vi "RunTest.vi"(8 "error in (no error)":errorcluster, 11 "TestCaseMock in":refnum<class "TestCaseMock.lvclass">) -> (0 "error out":errorcluster, 3 "TestCaseMock out":refnum<class "TestCaseMock.lvclass">)   [LabVIEW 2017, in "TestResultTest.lvlib" / "Support.lvlib" / "TestCaseMock.lvclass"]
doc: "Override to run the test and assert its state."
uses:
  TestCaseMock.lvclass
  Error/Error.lvlib
  a4c9ca4c-822c-43fa-bc73-5b07c458682f.vi
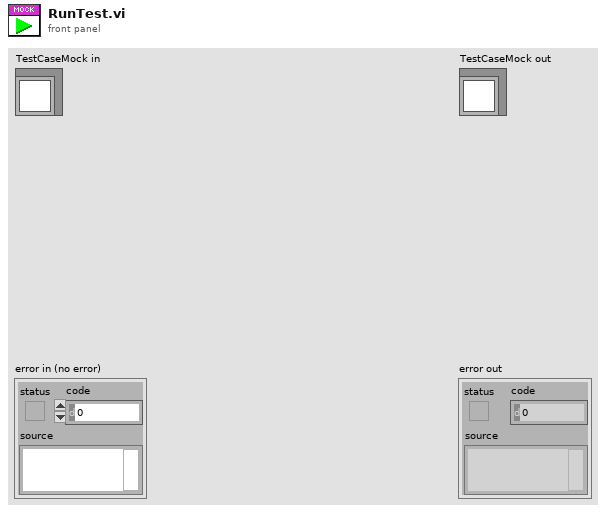
[diagram p1: front panel]
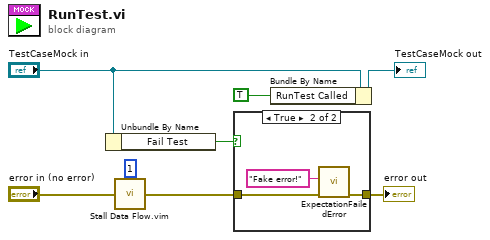
[diagram p0: block diagram]
diagram:
  n1 = Unbundle By Name("TestCaseMock in") -> ("Fail Test"=w3:bool)
  n2 = call "Stall Data Flow.vim"("value in"="error in (no error)", "milliseconds to wait"=u32 1) -> ("value out"=w2:errorcluster)  [unwired: 1 out]
  n3 = case shown="True" w3 {
    tunnel: w2 -> [w9 w11]
    tunnel: [w9 w12] -> w4
    frame False {
    }
    frame True {
      n4 = call "ExpectationFailedError.vi"("error in (no error)"=w11, "Message"="Fake error!") -> ("error out"=w12:errorcluster)  [unwired: 9 in]
    }
  }
  "error out" <- w4
  n5 = Bundle By Name(cluster="TestCaseMock in", "RunTest Called"=TRUE ("RunBare Called")) -> (→"TestCaseMock out":refnum<class "TestCaseMock.lvclass">)
